vi "Get_Access_Scope.vi"(8 "error in (no error)":errorcluster, 11 "AB_Source in":refnum<class "AB_Source.lvclass">) -> (0 "error out":errorcluster, 2 "Source Scope":T1(ring), 3 "AB_Source out":refnum<class "AB_Source.lvclass">)   [LabVIEW 2020, in "AB_Source.lvclass"]
uses:
  <vilib>/AppBuilder/AB_Classes/Source/AB_Source.lvclass
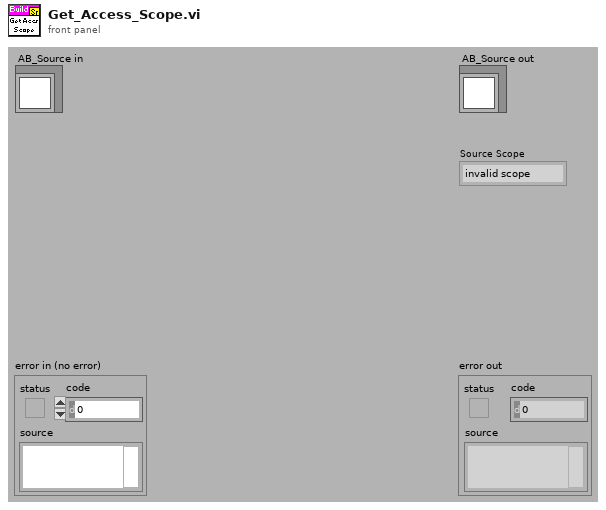
[diagram p1: front panel]
types:
  T1 = enum32{"invalid scope", "public", "private", "protected", "community"}
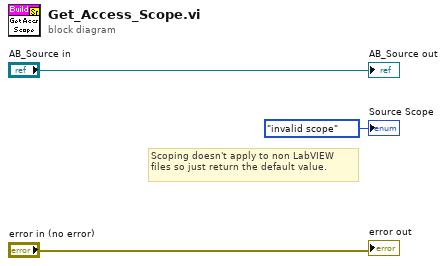
[diagram p0: block diagram]
diagram:
  # "Scoping doesn't apply to non LabVIEW files so just return the default value."
  "error out" <- "error in (no error)"
  "AB_Source out" <- "AB_Source in"
  "Source Scope" <- T1."invalid scope" ("Source Scope:Get")
